vi "KH_DAQ_WriteAll.vi"(6 "Numeric":i32, 8 "err in":errorcluster caption="error", 10 "EIP_AO":T1 {"Offset" format="%.4f"; "Phys Max" format="%.4f"; "Phys Min" format="%.4f"}, 11 "Output_IOL":T5={"IOL Port 1"=[0, 1], "IOL Port 2"=[0, 1], "IOL Port 3"=[0, 1], "IOL Port 4"=[0, 1]}) -> (0 "err out":errorcluster caption="error")   [LabVIEW 2021]
uses:
  KH_DAQ_TypeDefs_Cluster AO.ctl
  KH_DAQ_TypeDefs_Messbereich.ctl
  KH EthernetIPConfig 17.14/KH EthernetIPConfig TypeDefs ModuleTyp.ctl
  KH_DAQ_TypeDefs_Bereich.ctl
  KH Turck EthernetIP 17.12/KH TURCK TypeDefs FGlob.ctl
  KH Turck EthernetIP 17.12/KH TURCK ETHERNETIP TDefCluster TBEN-S1-8DXP Output Values.ctl
  KH EthernetIP 17.19/KH_EthernetIP_Globals.vi
  KH Turck EthernetIP 17.12/KH TURCK ETHERNETIP RFID ST READ Global.vi
  KH Turck EthernetIP 17.12/KH TURCK ETHERNETIP RFID Global.vi
  KH Turck EthernetIP 17.12/KH TURCK ETHERNETIP Global.vi
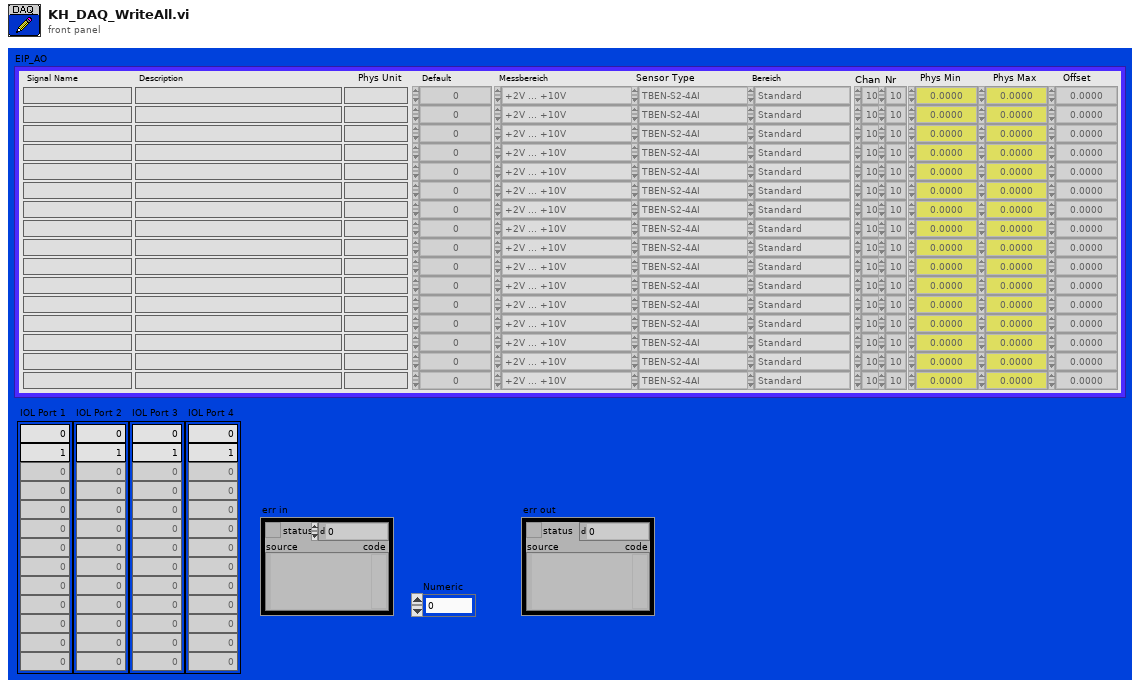
[diagram p1: front panel]
types:
  T1 = typedef "KH_DAQ_TypeDefs_Cluster AO.ctl" = cluster{"Signal Name":string[], "Description":string[], "Phys Unit":string[], "Messbereich":T2[], "Chan":u16[], "Phys Min":sgl[], "Phys Max":sgl[], "Offset":sgl[], "Nr":u16[], "SensorType 2":T3[], "Bereich":T4[], "Default":sgl[]}
  T2 = typedef "KH_DAQ_TypeDefs_Messbereich.ctl" = enum16{"-10V ... +10V", "0V ... +10V", "+2V ... +10V", "0V ... +5V", "+1V ... +5V", "-1V ... +1V", "-500mV ... +500mV", "-100mV ... +100mV", "-50mV ... +50mV", "0mA ... +20mA", "+4mA ... +20mA", "-20mA ... +20mA", "0 Ohm ... 100 Ohm", "0 Ohm ... 400 Ohm", "0 Ohm ... 2000 Ohm", "0 Ohm ... 4000 Ohm", "-200°C ... 150°C PT100", "-200°C ... 150°C PT200", "-200°C ... 150°C PT500", "-200°C ... 150°C PT1000", "-60°C ... 150°C Ni100", "-60°C ... 150°C Ni1000", "-200°C ... 850°C PT100", "-200°C ... 850°C PT200", "-200°C ... 850°C PT500", "-200°C ... 850°C PT1000", "-50°C ... 250°C Ni100", "-50°C ... 250° Ni 1000"}
  T3 = typedef "KH EthernetIPConfig TypeDefs ModuleTyp.ctl" = enum16{"TBEN-S2-4AI", "TBEN-S1-8DXP", "TBEN-S2-2RFID-4DXP", "TBEN-S2-4AO", "TBEN-S2-4IOL"}
  T4 = typedef "KH_DAQ_TypeDefs_Bereich.ctl" = enum16{"Standard", "extended Range", "NE43", ""}
  T5 = cluster{"IOL Port 1":u16[], "IOL Port 2":u16[], "IOL Port 3":u16[], "IOL Port 4":u16[]}
  T6 = typedef "KH EthernetIPConfig TDef Config.ctl" = cluster{"Typ":T3, "Name":string, "Nr.":i32, "InputOutput":enum16{"Input", "Output"}[]}
  T7 = typedef "KH TURCK TypeDefs FGlob.ctl" = enum16{"Put one", "Put all", "Recall one", "Recall all"}
  T8 = typedef "KH TURCK ETHERNETIP TDefCluster TBEN-S1-8DXP Output Values.ctl" = cluster{"Output Values":bool[], "Latch Resets":bool[], "Counter Reset":bool, "Duty Cycle Dig 3":u8, "Duty Cycle Dig 7":u8}
  T9 = typedef "KH TURCK ETHERNETIP TDef Enum RFID Data RFID.ctl" = cluster{"ResponseCode":u16, "LoopCounter":u8, "Length":u16, "WriteFragmentNo":u8, "ReadFragmentNo":u8, "Data":u8[], "TagPresent":bool, "Error":bool, "BusyFinished":bool, "Channel":u16}
  T10 = typedef "KH TURCK ETHERNETIP TDefCluster TURCK RFID.ctl" = cluster{"NumberOfBytes":i32, "State":string, "Counter":i32, "ReadData":u8[], "AnzahlFragmente":i32, "WritingFinished":bool, "ReadingFinished":bool, "UID":u8[], "ActCommand":T11, "SizeFragmentRead":i32, "LengthUID":u16, "WriteDataInclUID":u8[], "Timeout":bool, "SizeFragmentWrite":i32}
  T11 = typedef "KH TURCK ETHERNETIP TDef Enum RFID Act Command.ctl" = enum16{"read", "write", "idle", "Inventory", ""}
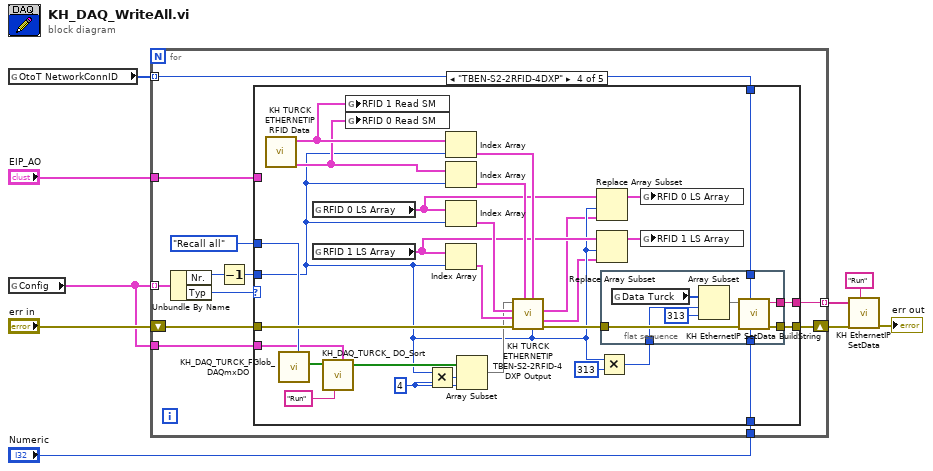
[diagram p0: block diagram]
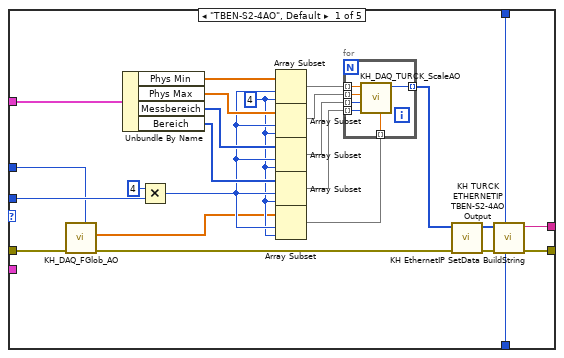
[diagram p2: hidden frame]
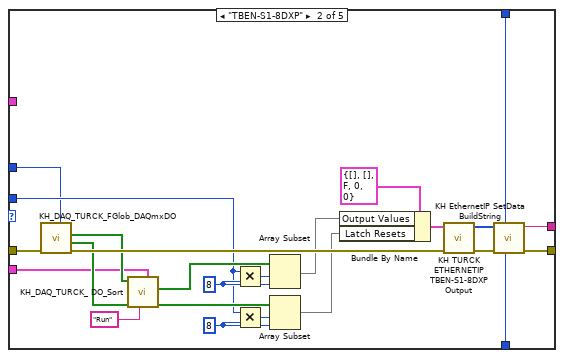
[diagram p3: hidden frame]
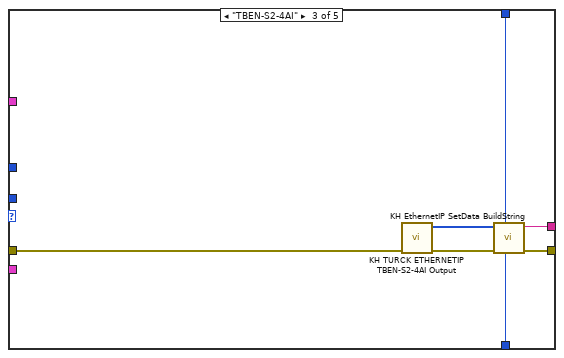
[diagram p4: hidden frame]
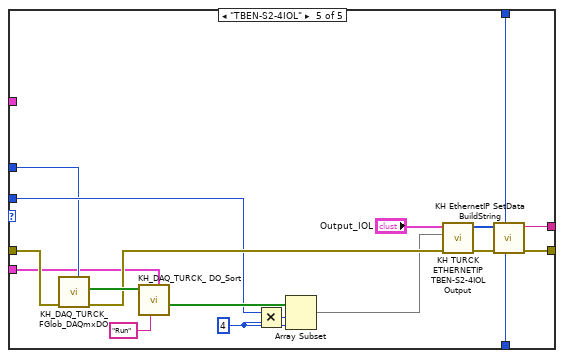
[diagram p5: hidden frame]
diagram:
  n1 = global read "KH_EthernetIP_Globals.vi" "OtoT NetworkConnID"() -> (w4:u32[])
  n2 = global read "KH_EthernetIP_Globals.vi" "Config"() -> (w3:T6[])
  n3 = for {
    tunnel: [w20] -> w8 mode=indexing
    shift-right: [w21] -> w9
    shift-left: "err in" -> [w19]
    tunnel: w4 -> [w17] mode=indexing
    tunnel: w3 -> [w16] mode=indexing
    tunnel: w3 -> [w13]
    tunnel: "EIP_AO" -> [w12]
    tunnel: "Numeric" -> [w10]
    n4 = Unbundle By Name(w16) -> ("Nr."=w15:i32, "Typ"=w18:T3)
    n5 = Decrement(x=w15) -> (x-1=w14:i32)
    n6 = case shown="\"TBEN-S2-2RFID-4DXP\"" w18 {
      tunnel: [w25 w73 w81 w112 w137] -> w21
      tunnel: w19 -> [w41 w68 w83 w104 w132]
      tunnel: [w24 w71 w79 w111 w136] -> w20
      tunnel: w10 -> [w45 w70 w78 w85 w135]
      tunnel: w17 -> [w43 w69 w77 w110 w134]
      tunnel: w14 -> [w31 w58 _ w88 w127]
      tunnel: w12 -> [w33 _ _ _ _]
      tunnel: w13 -> [_ w55 _ w91 w123]
      tunnel: KH_TURCK_TypeDefs_FGlob."Recall all" ("Function (Recall One)") -> [w22 w56 _ w92 w124]
      frame "TBEN-S2-4AO", Default {
        w30 = 4 ("length")
        n7 = call "KH_DAQ_FGlob_AO.vi"("Function (Recall One)"=w22, "err in"=w41) -> ("err out"=w40:errorcluster, "AO Values OUT"=w23:sgl[])  [unwired: 7 in, 1 out]
        n8 = Unbundle By Name(w33) -> ("Phys Min"=w36:sgl[], "Phys Max"=w37:sgl[], "Messbereich"=w38:T2[], "Bereich"=w39:T4[])
        n9 = Multiply(x=4, y=w31) -> (x*y=w32:i32)
        n10 = Array Subset(array=w36, index=w32, length=w30) -> (w35:sgl[])
        n11 = Array Subset(array=w37, index=w32, length=w30) -> (w34:sgl[])
        n12 = Array Subset(array=w38, index=w32, length=w30) -> (w29:T2[])
        n13 = Array Subset(array=w39, index=w32, length=w30) -> (w28:T4[])
        n14 = Array Subset(array=w23, index=w32, length=w30) -> (w27:sgl[])
        n15 = for {
          tunnel: w35 -> [w52] mode=indexing
          tunnel: w34 -> [w51] mode=indexing
          tunnel: w28 -> [w47] mode=indexing
          tunnel: [w50] -> w26 mode=indexing
          tunnel: w29 -> [w49] mode=indexing
          tunnel: w27 -> [w48] mode=indexing
          n16 = call "KH_DAQ_TURCK_ScaleAO.vi"("Sollwert"=w48, "Bereich"=w47, "Messbereich"=w49, "PhysMax"=w51, "PhysMin"=w52) -> ("Sollwert Turck"=w50:i16)  [unwired: 6 in]
        }
        n17 = call "KH TURCK ETHERNETIP TBEN-S2-4AO Output.vi"("error in"=w40, "TBEN-S2-4AO Output Values"=w26) -> ("error out"=w46:errorcluster, "Output Data"=w44:u8[])  [unwired: 8 in]
        n18 = call "KH EthernetIP SetData BuildString.vi"("LoopIndex"=w45, "OtoT NetworkConnID"=w43, "error in"=w46, "Output Data"=w44) -> ("error out"=w25:errorcluster, "DataString"=w24:string)  [unwired: 6 in]
      }
      frame "TBEN-S1-8DXP" {
        w61 = 8 ("length")
        w65 = 8 ("length")
        n19 = call "KH_DAQ_TURCK_FGlob_DAQmxDO.vi"("Function (Recall One)"=w56, "err in"=w68) -> ("err out"=w67:errorcluster, "DXP Reset OUT"=w60:bool[], "DXP Values OUT"=w66:bool[])  [unwired: 6 in, 1 out]
        n20 = call "KH_DAQ_TURCK_ DO_Sort.vi"("Config"=w55, "Function"="Run", "ResetDXP"=w60, "DOs"=w66) -> ("DXP Reset"=w59:bool[], "DO_DXP"=w63:bool[])  [unwired: 4 in, 2 out]
        n21 = Multiply(x=w58, y=w65) -> (x*y=w64:i32)
        n22 = Multiply(x=w58, y=w61) -> (x*y=w53:i32)
        n23 = Array Subset(array=w63, index=w64, length=w65) -> (w62:bool[])
        n24 = Array Subset(array=w59, index=w53, length=w61) -> (w57:bool[])
        n25 = Bundle By Name(cluster=T8 {"Output Values"=[], "Latch Resets"=[], "Counter Reset"=FALSE, "Duty Cycle Dig 3"=0, "Duty Cycle Dig 7"=0} ("TBEN-S1-8DXP Output Values"), "Output Values"=w62, "Latch Resets"=w57) -> (w75:T8)
        n26 = call "KH TURCK ETHERNETIP TBEN-S1-8DXP Output.vi"("error in"=w67, "TBEN-S1-8DXP Output Values"=w75) -> ("error out"=w74:errorcluster, "Output Data"=w72:u8[])  [unwired: 8 in]
        n27 = call "KH EthernetIP SetData BuildString.vi"("LoopIndex"=w70, "OtoT NetworkConnID"=w69, "error in"=w74, "Output Data"=w72) -> ("error out"=w73:errorcluster, "DataString"=w71:string)  [unwired: 6 in]
      }
      frame "TBEN-S2-4AI" {
        n28 = call "KH TURCK ETHERNETIP TBEN-S2-4AI Output.vi"("error in"=w83) -> ("error out"=w80:errorcluster, "Output Data"=w82:u8[])  [unwired: 9 in]
        n29 = call "KH EthernetIP SetData BuildString.vi"("LoopIndex"=w78, "OtoT NetworkConnID"=w77, "error in"=w80, "Output Data"=w82) -> ("error out"=w81:errorcluster, "DataString"=w79:string)  [unwired: 6 in]
      }
      frame "TBEN-S2-2RFID-4DXP" {
        w102 = 4 ("length")
        n30 = call "KH TURCK ETHERNETIP RFID Data.vi"() -> ("RFID 0 Read SM"=w89:T9[], "RFID 1 Read SM"=w90:T9[])  [unwired: 10 in]
        n31 = call "KH_DAQ_TURCK_FGlob_DAQmxDO.vi"("Function (Recall One)"=w92) -> ("DXP Values OUT"=w103:bool[])  [unwired: 7 in, 3 out]
        n32 = global read "KH TURCK ETHERNETIP RFID Global.vi" "RFID 0 LS Array"() -> (w94:T10[])
        n33 = global read "KH TURCK ETHERNETIP RFID Global.vi" "RFID 1 LS Array"() -> (w97:T10[])
        n34 = call "KH_DAQ_TURCK_ DO_Sort.vi"("Config"=w91, "Function"="Run", "DOs"=w103) -> ("DO_RFID"=w100:bool[])  [unwired: 5 in, 3 out]
        n35 = global write "KH TURCK ETHERNETIP RFID ST READ Global.vi" "RFID 1 Read SM"(w90) -> ()
        n36 = global write "KH TURCK ETHERNETIP RFID ST READ Global.vi" "RFID 0 Read SM"(w89) -> ()
        n37 = Multiply(x=w88, y=w102) -> (x*y=w101:i32)
        n38 = Index Array(array=w90, index=w88) -> (element=w108:T9)
        n39 = Index Array(array=w89, index=w88) -> (element=w107:T9)
        n40 = Index Array(array=w94, index=w88) -> (element=w106:T10)
        n41 = Index Array(array=w97, index=w88) -> (element=w105:T10)
        n42 = Array Subset(array=w100, index=w101, length=w102) -> (w93:bool[])
        n43 = call "KH TURCK ETHERNETIP TBEN-S2-2RFID-4DXP Output.vi"("Nr Modul"=w88, "Read 1 SM"=w108, "Read 0 SM"=w107, "error in"=w104, "ReadWrite 1 SM In"=w105, "ReadWrite 0 SM In"=w106, "RFID DXP"=w93) -> ("error out"=w109:errorcluster, "ReadWrite 1 SM Out"=w86:T10, "ReadWrite 0 SM Out"=w87:T10)  [unwired: 1 in, 1 out]
        n44 = Replace Array Subset(array=w94, new element=w87, index=w88) -> (w95:T10[])
        n45 = Replace Array Subset(array=w97, new element=w86, index=w88) -> (w96:T10[])
        n46 = Multiply(x=w88, y=313) -> (x*y=w98:i32)
        n47 = flat-sequence {
          tunnel: [w121] -> w112
          tunnel: w110 -> [w120]
          tunnel: [w119] -> w111
          tunnel: w85 -> [w118]
          tunnel: w109 -> [w116]
          tunnel: w98 -> [w114]
          frame #0 {
            n48 = global read "KH TURCK ETHERNETIP Global.vi" "Data Turck"() -> (w113:u8[])
            n49 = Array Subset(array=w113, index=w114, length=313) -> (w115:u8[])
            n50 = call "KH EthernetIP SetData BuildString.vi"("LoopIndex"=w118, "OtoT NetworkConnID"=w120, "error in"=w116, "Output Data"=w115) -> ("error out"=w121:errorcluster, "DataString"=w119:string)  [unwired: 6 in]
          }
        }
        n51 = global write "KH TURCK ETHERNETIP RFID Global.vi" "RFID 0 LS Array"(w95) -> ()
        n52 = global write "KH TURCK ETHERNETIP RFID Global.vi" "RFID 1 LS Array"(w96) -> ()
      }
      frame "TBEN-S2-4IOL" {
        w130 = 4 ("length")
        n53 = call "KH_DAQ_TURCK_FGlob_DAQmxDO.vi"("Function (Recall One)"=w124, "err in"=w132) -> ("err out"=w131:errorcluster, "DXP Values OUT"=w133:bool[])  [unwired: 6 in, 2 out]
        n54 = call "KH_DAQ_TURCK_ DO_Sort.vi"("Config"=w123, "Function"="Run", "DOs"=w133) -> ("DO_IOL"=w128:bool[])  [unwired: 5 in, 3 out]
        n55 = Multiply(x=w127, y=w130) -> (x*y=w129:i32)
        n56 = Array Subset(array=w128, index=w129, length=w130) -> (w125:bool[])
        n57 = call "KH TURCK ETHERNETIP TBEN-S2-4IOL Output.vi"("error in"=w131, "DXP"=w125, "Output_IOL"="Output_IOL") -> ("error out"=w138:errorcluster, "Output Data"=w139:u8[])  [unwired: 7 in]
        n58 = call "KH EthernetIP SetData BuildString.vi"("LoopIndex"=w135, "OtoT NetworkConnID"=w134, "error in"=w138, "Output Data"=w139) -> ("error out"=w137:errorcluster, "DataString"=w136:string)  [unwired: 6 in]
      }
    }
  }
  n59 = call "KH EthernetIP SetData.vi"("Function"="Run", "error in"=w9, "Data Strings"=w8) -> ("error out"=→"err out":errorcluster)  [unwired: 6 in, 2 out]
